vi "3byte转换.vi"(11 "字符串":string) -> (3 "数值":i32)   [LabVIEW 2023]
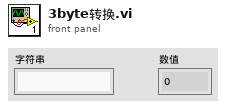
[diagram p1: front panel]
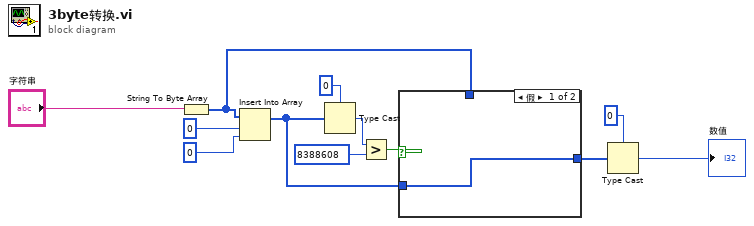
[diagram p0: block diagram]
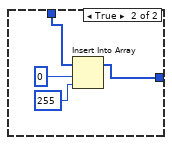
[diagram p2: hidden frame]
diagram:
  n1 = String To Byte Array(string="字符串") -> (unsigned byte array=w8:u8[])
  n2 = Insert Into Array(array=w8, index=0 ("索引"), new element=u8 0 ("新元素/子数组")) -> (w11:u8[])
  n3 = Type Cast(type=0 ("索引"), x=w11) -> (*(type *) &x=w5:i32)
  n4 = Greater?(x=w5, y=8388608) -> (0:w7:bool)
  n5 = case shown="假" w7 {
    tunnel: w8 -> [_ w17]
    tunnel: [w13 w14] -> w10
    tunnel: w11 -> [w13 _]
    frame False {
    }
    frame True {
      n6 = Insert Into Array(array=w17, index=0 ("索引"), new element=u8 255 ("新元素/子数组")) -> (w14:u8[])
    }
  }
  n7 = Type Cast(type=0, x=w10) -> (*(type *) &x=→"数值":i32)
